vi "PDE String Vibration.vi"() -> ()   [LabVIEW 2023]
doc: "This example demonstrates how to use the Partial Differential Equations VIs to define and solve a 1-dimensional wave equation. Suppose that there is a string with both ends fixed. If it is displaced from the equilibrium position and released, the string starts vibration. The 1-dimensional wave equation in this example describes the ideal vibration as time evolves."
uses:
  <vilib>/gmath/pde.llb/Common/PDE_BC Type.ctl
  <vilib>/gmath/pde.llb/Common/PDE_BC Position 1D.ctl
  <vilib>/gmath/pde.llb/Common/PDE_IC Type.ctl
  <vilib>/Analysis/1siggen.llb/Ramp Pattern by Samples.vi
  <vilib>/gmath/pde.llb/Define 1D Wave PDE (Numeric).vi
  <vilib>/gmath/pde.llb/Define 1D Wave PDE Domain.vi
  <vilib>/gmath/pde.llb/Define 1D Wave PDE BC (Numeric).vi
  <vilib>/gmath/pde.llb/Define 1D Wave PDE IC (VIRef).vi
  <vilib>/gmath/pde.llb/Define 1D Wave PDE IC (Numeric).vi
  <vilib>/gmath/pde.llb/1D Wave PDE Solver.vi
  <vilib>/gmath/pde.llb/1D Wave PDE Rendering.vi
  <vilib>/gmath/NI_PDE.lvlib
  <vilib>/Analysis/NI_AALBase.lvlib
panel:
  in  "Stop":bool
  out "Displacement over Time":dbl[][](graph)
  out "String Vibration":cluster{"Ramp Pattern":dbl[], "U(t, x)":dbl[]}[](graph)
  in  "Initial Position":dbl(slide)=0.6 min=0.2 max=0.8 step=0.01 scale=0.2..0.8 scale format="%#.2g"
  out "Current Time (s)":dbl(slide) scale=0.0..10.0
  # "Overview: This example demonstrates how to use the Partial Differential Equations VIs to define and solve a 1-dimensional wave equation.\nRequirements: LabVIEW Full Development System\nInstructions: \n1. Specify the Initial Position to define the vibration of the string.\n2. Run the VI.\n3. Click Stop to stop the VI."
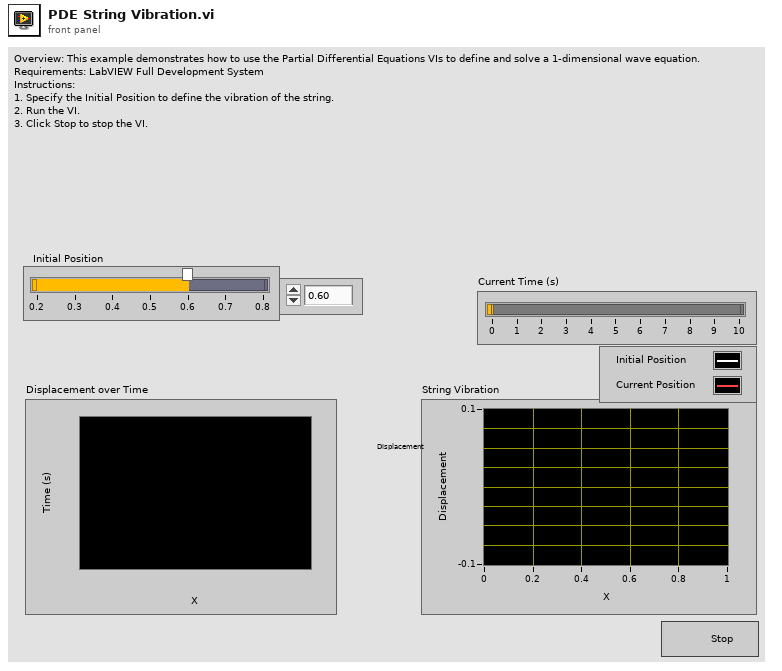
[diagram p1: front panel]
types:
  T1 = cluster{"start x":dbl, "end x":dbl, "# of x-points":i32}
  T2 = cluster{"initial t":dbl, "final t":dbl, "# of t-points":i32}
  T3 = typedef "NI_PDE.lvlib/PDE_BC Position 1D.ctl" = i32
  T4 = typedef "NI_PDE.lvlib/PDE_IC Type.ctl" = i32
  T5 = typedef "NI_PDE.lvlib/PDE_BC Type.ctl" = i32
  T6 = typedef "LVOffsetAndMultiplierTypeDef.ctl" = cluster{"Offset":dbl, "Multiplier":dbl}
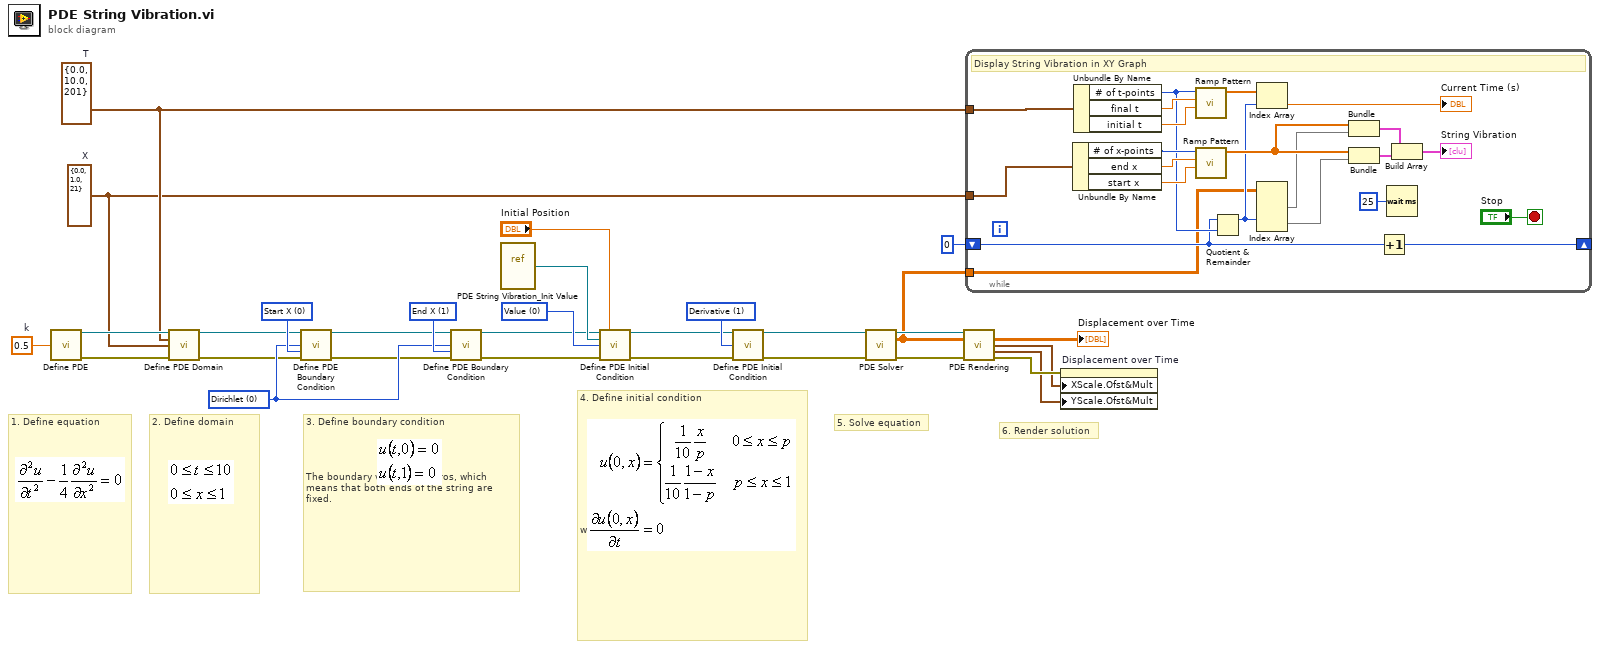
[diagram p0: block diagram]
diagram:
  w1 = T1 {"start x"=0.0, "end x"=1.0, "# of x-points"=21}  # X
  w2 = T2 {"initial t"=0.0, "final t"=10.0, "# of t-points"=201}  # T
  w28 = 0.5  # k
  w24 = T3 1 items=["Start X", "End X"] ("position")
  w22 = T4 1 items=["Value", "Derivative"] ("type")
  w17 = T4 0 items=["Value", "Derivative"] ("type")
  w14 = T3 0 items=["Start X", "End X"] ("position")
  w13 = T5 0 items=["Dirichlet", "Neumann"] ("type")
  # "6. Render solution"
  # "5. Solve equation"
  # "4. Define initial condition\n\n\n\n\n\n\n\n\n\n\n\nwhere p is specified by Initial Position."
  # "3. Define boundary condition\n\n\n\n\nThe boundary values are zeros, which means that both ends of the string are fixed."
  # "2. Define domain"
  # "1. Define equation"
  n1 = call-poly <vilib>:"Define PDE.vi"("k"=w28) -> ("PDE out"=w5:refnum<class "NI_PDE.lvclass">, "error out"=w8:errorcluster)  [unwired: 4 in, 9 out]
  n2 = call-poly <vilib>:"Define PDE Domain.vi"("PDE in"=w5, "T"=w2, "X"=w1, "error in (no error)"=w8) -> ("PDE out"=w6:refnum<class "NI_PDE.lvclass">, "error out"=w7:errorcluster)  [unwired: 10 out]
  n3 = call-poly <vilib>:"Define PDE Boundary Condition.vi"("PDE in"=w6, "type"=w13, "position"=w14, "error in (no error)"=w7) -> ("PDE out"=w11:refnum<class "NI_PDE.lvclass">, "error out"=w12:errorcluster)  [unwired: 1 in, 9 out]
  n4 = call-poly <vilib>:"Define PDE Boundary Condition.vi"("PDE in"=w11, "type"=w13, "position"=w24, "error in (no error)"=w12) -> ("PDE out"=w15:refnum<class "NI_PDE.lvclass">, "error out"=w16:errorcluster)  [unwired: 1 in, 9 out]
  n5 = vi-ref "PDE String Vibration_Init Value.vi"() -> (w29:refnum<vi>)
  n6 = call-poly <vilib>:"Define PDE Initial Condition.vi"("PDE in"=w15, "data"="Initial Position", "Initial Condition"=w29, "type"=w17, "error in (no error)"=w16) -> ("PDE out"=w21:refnum<class "NI_PDE.lvclass">, "error out"=w18:errorcluster)  [unwired: 9 out]
  n7 = call-poly <vilib>:"Define PDE Initial Condition.vi"("PDE in"=w21, "type"=w22, "error in (no error)"=w18) -> ("PDE out"=w20:refnum<class "NI_PDE.lvclass">, "error out"=w19:errorcluster)  [unwired: 1 in, 10 out]
  n8 = call-poly <vilib>:"PDE Solver.vi"("PDE in"=w20, "error in (no error)"=w19) -> ("PDE out"=w9:refnum<class "NI_PDE.lvclass">, "U(t, x)"=w3:dbl[][], "error out"=w10:errorcluster)  [unwired: 11 out]
  n9 = call-poly <vilib>:"PDE Rendering.vi"("PDE in"=w9, "U(t, x)"=w3, "error in (no error)"=w10) -> ("PDE Plot"=→"Displacement over Time":dbl[][], "X Scale"=w25:T6, "Y Scale"=w26:T6, "error out"=w27:errorcluster)  [unwired: 9 out]
  n10 = while {
    shift-right: [w31] -> _
    shift-left: 0 -> [w37]
    tunnel: w2 -> [w33]
    tunnel: w1 -> [w32]
    tunnel: w3 -> [w36]
    stop <- "Stop" stop-if-true
    # "Display String Vibration in XY Graph"
    n11 = Unbundle By Name(w32) -> ("# of x-points"=w52:i32, "end x"=w51:dbl, "start x"=w50:dbl)
    n12 = Unbundle By Name(w33) -> ("# of t-points"=w43:i32, "final t"=w45:dbl, "initial t"=w46:dbl)
    n13 = call-poly <vilib>:"Ramp Pattern.vi"("start"=w46, "end"=w45, "samples"=w43) -> ("Ramp Pattern"=w44:dbl[])  [unwired: 7 in, 1 out]
    n14 = call-poly <vilib>:"Ramp Pattern.vi"("start"=w50, "end"=w51, "samples"=w52) -> ("Ramp Pattern"=w49:dbl[])  [unwired: 7 in, 1 out]
    n15 = Quotient & Remainder(x=w37, y=w43) -> (x-y*floor(x/y)=w38:i32)  [unwired: 1 out]
    n16 = Index Array(array=w44, index=w38) -> (element=→"Current Time (s)":dbl)
    n17 = Index Array(array=w36, index (row) #2=w38) -> (element #1=w48:dbl[], element #2=w39:dbl[])  [unwired: 3 in]
    n18 = Bundle("Ramp Pattern"=w49, "U(t, x)"=w48) -> (w47:cluster{"Ramp Pattern":dbl[], "U(t, x)":dbl[]})  [unwired: 1 out]
    n19 = Bundle("Ramp Pattern"=w49, "U(t, x)"=w39) -> (w42:cluster{"Ramp Pattern":dbl[], "U(t, x)":dbl[]})  [unwired: 1 out]
    n20 = Increment(x=w37) -> (x+1=w31:i32)
    n21 = Wait (ms)(milliseconds to wait=u32 25) -> ()  [unwired: 1 out]
    n22 = Build Array(w47, w42) -> (→"String Vibration":cluster{"Ramp Pattern":dbl[], "U(t, x)":dbl[]}[])
  }
  n23 = property on="Displacement over Time" class="IntGraph (strict)"(error in=w27, "XScale.Ofst&Mult"=w25, "YScale.Ofst&Mult"=w26) -> ()  [unwired: 1 in, 2 out]
